vi "Read Counter Driven Output Channel.vi"(8 "error in":errorcluster, 11 "counter driven output channel in":refnum<class "Counter Driven Output Channel.lvclass">) -> (0 "error out":errorcluster, 1 "default value":bool, 2 "name":string, 3 "counter driven output channel out":refnum<class "Counter Driven Output Channel.lvclass">, 4 "index":i32, 5 "counter driven state":T1)   [LabVIEW 2020, in "Scan Engine Scripting.lvlib" / "Counter Driven Output Channel.lvclass"]
uses:
  Counter Driven Output Channel.lvclass
  Counter Driven State.ctl
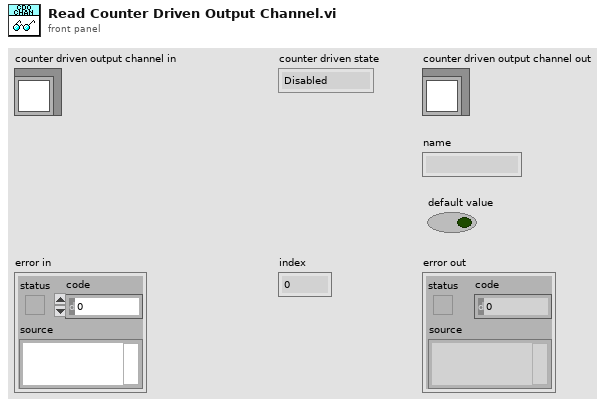
[diagram p1: front panel]
types:
  T1 = typedef "Scan Engine Scripting.lvlib/Counter Driven Output Channel.lvclass/Counter Driven State.ctl" = enum16{"Disabled", "Enabled"}
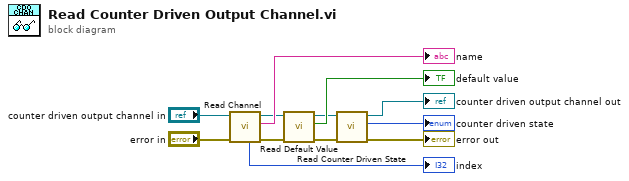
[diagram p0: block diagram]
diagram:
  n1 = call-dynamic "Read Channel.vi"("error in"="error in", "channel in"="counter driven output channel in") -> ("error out"=w2:errorcluster, "name"=→"name":string, "channel out"=w4:refnum<class "Counter Driven Output Channel.lvclass">, "index"=→"index":i32)  [unwired: 4 in, 2 out]
  n2 = call-dynamic "Read Default Value.vi"("error in"=w2, "digital channel in"=w4) -> ("error out"=w1:errorcluster, "default value"=→"default value":bool, "digital channel out"=w3:refnum<class "Counter Driven Output Channel.lvclass">)  [unwired: 7 in]
  n3 = call-dynamic "Read Counter Driven State.vi"("error in"=w1, "counter driven output channel in"=w3) -> ("error out"=→"error out":errorcluster, "counter driven state"=→"counter driven state":T1, "counter driven output channel out"=→"counter driven output channel out":refnum<class "Counter Driven Output Channel.lvclass">)  [unwired: 7 in]
